vi "OpenPump.vi"(11 "VISA Refnum in":refnum<visa-resource-name>="COM4") -> (0 "error out":errorcluster, 3 "VISA Refnum out":refnum<visa-resource-name>)   [LabVIEW 2020]
uses:
  <vilib>/Instr/_visa.llb/VISA Configure Serial Port (Instr).vi
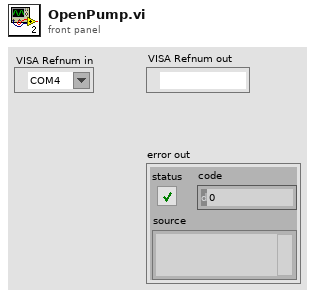
[diagram p1: front panel]
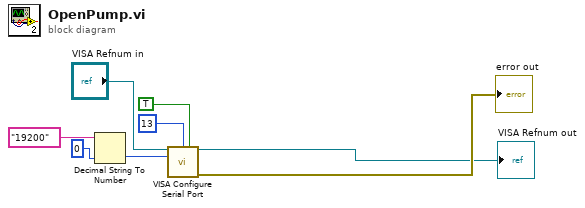
[diagram p0: block diagram]
diagram:
  n1 = Decimal String To Number(string="19200" ("Baud Rate"), default (0L)=u32 0 ("default (0 I32)")) -> (number=w5:u32)  [unwired: 1 in, 1 out]
  n2 = call-poly "VISA Configure Serial Port"("VISA resource name"="VISA Refnum in", "termination char\n(0xA = '\\n' = LF)"=u8 13 ("termination char\n(0xA = '\\n' = LF)"), "Enable Termination\nChar (T)"=TRUE ("Enable Termination\nChar (T)"), "baud rate (9600)"=w5) -> ("VISA resource name out"=→"VISA Refnum out":refnum<visa-resource-name>, "error out"=→"error out":errorcluster)  [unwired: 10 in]
